vi "MListbox Replace Cell.vi"(6 "Backcolor":u32(colorbox)=16448250, 8 "error in (no error)":errorcluster, 9 "String":string, 10 "index":cluster{"Row":u16, "Colunm":u16}, 11 "Multicolumn ListBox in":refnum<class "Multicolumn ListBox.lvclass">) -> (0 "error out":errorcluster, 3 "Multicolumn ListBox out":refnum<class "Multicolumn ListBox.lvclass">)   [LabVIEW 2012, in "Multicolumn ListBox.lvclass"]
uses:
  Multicolumn ListBox.lvclass
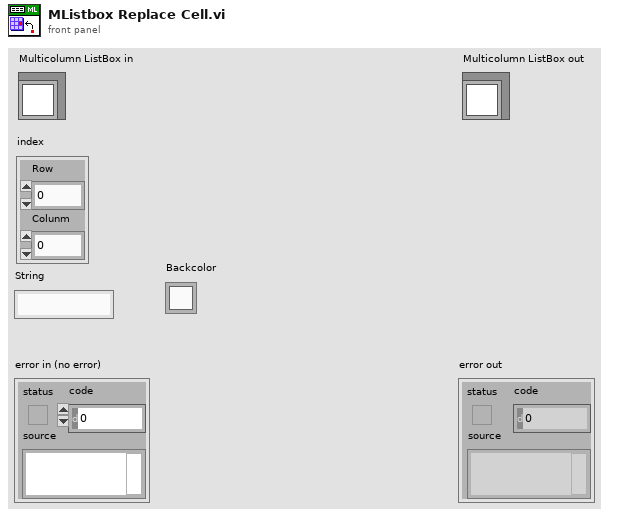
[diagram p1: front panel]
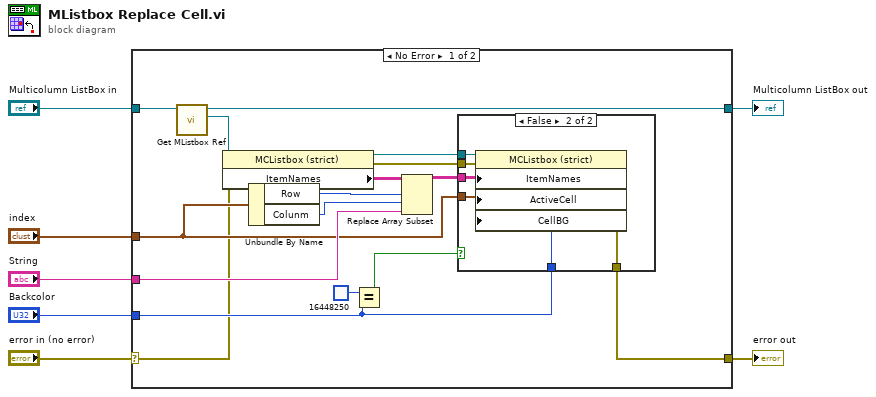
[diagram p0: block diagram]
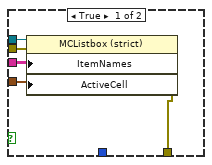
[diagram p2: hidden frame]
diagram:
  n1 = case shown="No Error" "error in (no error)" {
    selector: "error in (no error)" -> [w9 w36]
    tunnel: [w8 w36] -> w6
    tunnel: [w22 w35] -> w4
    tunnel: "Multicolumn ListBox in" -> [w23 w35]
    tunnel: "index" -> [w14 _]
    tunnel: "String" -> [w17 _]
    tunnel: "Backcolor" -> [w11 _]
    frame No Error {
      n2 = call "Get MListbox Ref.vi"("Multicolumn ListBox in"=w23) -> ("MListbox Ref"=w21:refnum<vi>, "Multicolumn ListBox out"=w22:refnum<class "Multicolumn ListBox.lvclass">)  [unwired: 8 in, 1 out]
      n3 = property class="MCListbox (strict)"(reference=w21, error in=w9) -> (reference out=w16:refnum<vi>, error out=w10:errorcluster, "ItemNames"=w20:string[][])
      n4 = Unbundle By Name(w14) -> ("Row"=w19:u16, "Colunm"=w18:u16)
      n5 = Equal?(x=u32 16448250 ("Backcolor"), y=w11) -> (x = y?=w12:bool)
      n6 = Replace Array Subset(array=w20, new element=w17, index (row)=w19, index (col)=w18) -> (w15:string[][])
      n7 = case shown="False" w12 {
        tunnel: w16 -> [w28 w34]
        tunnel: w15 -> [w27 w33]
        tunnel: w14 -> [w26 w32]
        tunnel: w11 -> [_ w31]
        tunnel: w10 -> [w25 w30]
        tunnel: [w24 w29] -> w8
        frame True {
          n8 = property class="MCListbox (strict)"(reference=w28, error in=w25, "ItemNames"=w27, "ActiveCell"=w26) -> (error out=w24:errorcluster)  [unwired: 1 out]
        }
        frame False {
          n9 = property class="MCListbox (strict)"(reference=w34, error in=w30, "ItemNames"=w33, "ActiveCell"=w32, "CellBG"=w31) -> (error out=w29:errorcluster)  [unwired: 1 out]
        }
      }
    }
    frame Error {
    }
  }
  "error out" <- w6
  "Multicolumn ListBox out" <- w4
